vi "example_alignObjects2.vi"   [LabVIEW 2023]
uses:
  Ctrls/alignment.ctl
  BlockDiagram/BlockDiagram.lvclass
  C:/projects/TLC_Scripto/Source/AbstractDiagram/AbstractDiagram.lvclass
  Terminal/Terminal.lvclass
  C:/projects/TLC_Scripto/Source/GObject/GObject.lvclass
  AbstractDiagram/Read controlTerminals.vi
  GObject/GObject.lvclass
  TLC_Scripto.lvlib
types:
  T1 = typedef "TLC_Scripto.lvlib/alignment.ctl" = enum16{"Top", "Bottom", "Left", "Right", "Center"}
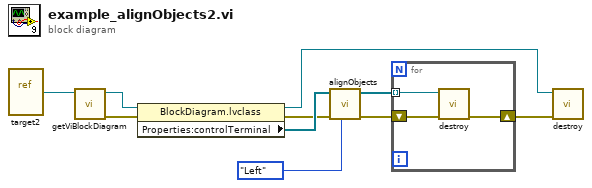
[diagram p0: block diagram]
diagram:
  n1 = vi-ref "target2.vi"() -> (w10:refnum<vi>)
  n2 = call "getViBlockDiagram.vi"("ViRef"=w10) -> ("error out"=w9:errorcluster, "topMostBlockDiagram"=w8:refnum<class "BlockDiagram.lvclass">)  [unwired: 9 in]
  n3 = property class="BlockDiagram.lvclass"(reference=w8, error in=w9) -> (reference out=w6:refnum<class "BlockDiagram.lvclass">, error out=w4:errorcluster, "Properties:controlTerminal"=w5:refnum<class "Terminal.lvclass">[])
  n4 = call "alignObjects.vi"("alignment"=alignment."Left", "error in (no error)"=w4, "GObjectsIn"=w5) -> ("error out"=w3:errorcluster, "GObjectsOut"=w1:refnum<class "GObject.lvclass">[])  [unwired: 7 in]
  n5 = for {
    shift-right: [w13] -> w7
    shift-left: w3 -> [w12]
    tunnel: w1 -> [w11] mode=indexing
    n6 = call-dynamic "destroy.vi"("Error In"=w12, "Generic In"=w11) -> ("Error Out"=w13:errorcluster)  [unwired: 9 in]
  }
  n7 = call-dynamic "destroy.vi"("Error In"=w7, "Generic In"=w6) -> ()  [unwired: 9 in, 1 out]
